vi "Convert SPI Data to Numbers.vi"(0 "Data In":bool[](array[boolean])) -> (1 "IBP Data":T1, 2 "ECG Data":T2)   [LabVIEW 2016]
uses:
  ECG Data.ctl
  IBP Data.ctl
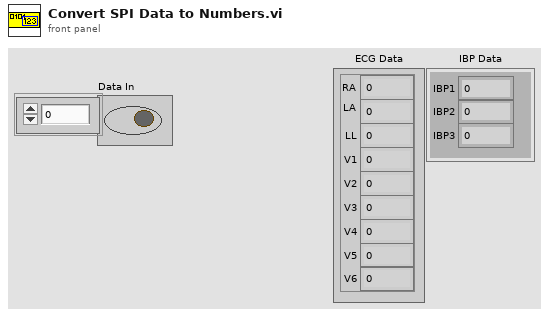
[diagram p1: front panel]
types:
  T1 = typedef "IBP Data.ctl" = cluster{"IBP1":fxp<+/-,16,16>, "IBP2":fxp<+/-,16,16>, "IBP3":fxp<+/-,16,16>}
  T2 = typedef "ECG Data.ctl" = cluster{"RA":fxp<+/-,16,16>, "LA":fxp<+/-,16,16>, "LL":fxp<+/-,16,16>, "V1":fxp<+/-,16,16>, "V2":fxp<+/-,16,16>, "V3":fxp<+/-,16,16>, "V4":fxp<+/-,16,16>, "V5":fxp<+/-,16,16>, "V6":fxp<+/-,16,16>}
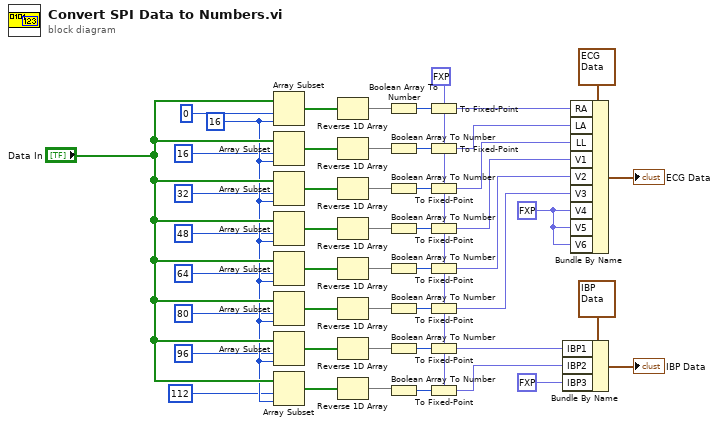
[diagram p0: block diagram]
diagram:
  w9 = fxp<+/-,16,16> 0.0 ("V4")
  w3 = fxp<+/-,16,16> 0.0 ("fixed-point type")
  w24 = 16 ("length")
  n1 = Array Subset(array="Data In", index=0, length=w24) -> (w34:bool[])
  n2 = Array Subset(array="Data In", index=16, length=w24) -> (w35:bool[])
  n3 = Array Subset(array="Data In", index=32, length=w24) -> (w36:bool[])
  n4 = Array Subset(array="Data In", index=48, length=w24) -> (w37:bool[])
  n5 = Array Subset(array="Data In", index=64, length=w24) -> (w38:bool[])
  n6 = Array Subset(array="Data In", index=80, length=w24) -> (w39:bool[])
  n7 = Array Subset(array="Data In", index=96, length=w24) -> (w40:bool[])
  n8 = Array Subset(array="Data In", index=112, length=w24) -> (w41:bool[])
  n9 = Reverse 1D Array(array=w34) -> (reversed array=w26:bool[])
  n10 = Reverse 1D Array(array=w35) -> (reversed array=w33:bool[])
  n11 = Reverse 1D Array(array=w36) -> (reversed array=w27:bool[])
  n12 = Reverse 1D Array(array=w37) -> (reversed array=w32:bool[])
  n13 = Reverse 1D Array(array=w38) -> (reversed array=w28:bool[])
  n14 = Reverse 1D Array(array=w39) -> (reversed array=w31:bool[])
  n15 = Reverse 1D Array(array=w40) -> (reversed array=w29:bool[])
  n16 = Reverse 1D Array(array=w41) -> (reversed array=w30:bool[])
  n17 = Boolean Array To Number(Boolean array=w26) -> (number=w43:i16)
  n18 = Boolean Array To Number(Boolean array=w33) -> (number=w44:i16)
  n19 = Boolean Array To Number(Boolean array=w27) -> (number=w45:i16)
  n20 = Boolean Array To Number(Boolean array=w32) -> (number=w46:i16)
  n21 = Boolean Array To Number(Boolean array=w28) -> (number=w47:i16)
  n22 = Boolean Array To Number(Boolean array=w31) -> (number=w48:i16)
  n23 = Boolean Array To Number(Boolean array=w29) -> (number=w7:i16)
  n24 = Boolean Array To Number(Boolean array=w30) -> (number=w6:i16)
  n25 = To Fixed-Point(fixed-point type=w3, number=w43) -> (fixed-point=w15:fxp<+/-,16,16>)
  n26 = To Fixed-Point(fixed-point type=w3, number=w44) -> (fixed-point=w14:fxp<+/-,16,16>)
  n27 = To Fixed-Point(fixed-point type=w3, number=w45) -> (fixed-point=w13:fxp<+/-,16,16>)
  n28 = To Fixed-Point(fixed-point type=w3, number=w46) -> (fixed-point=w12:fxp<+/-,16,16>)
  n29 = To Fixed-Point(fixed-point type=w3, number=w47) -> (fixed-point=w11:fxp<+/-,16,16>)
  n30 = To Fixed-Point(fixed-point type=w3, number=w48) -> (fixed-point=w10:fxp<+/-,16,16>)
  n31 = To Fixed-Point(fixed-point type=w3, number=w7) -> (fixed-point=w5:fxp<+/-,16,16>)
  n32 = To Fixed-Point(fixed-point type=w3, number=w6) -> (fixed-point=w4:fxp<+/-,16,16>)
  n33 = Bundle By Name(cluster=T1 {"IBP1"=0.0, "IBP2"=0.0, "IBP3"=0.0} ("IBP Data"), "IBP1"=w5, "IBP2"=w4, "IBP3"=fxp<+/-,16,16> 0.0) -> (→"IBP Data":T1)
  n34 = Bundle By Name(cluster=T2 {"RA"=0.0, "LA"=0.0, "LL"=0.0, "V1"=0.0, "V2"=0.0, "V3"=0.0, "V4"=0.0, "V5"=0.0, "V6"=0.0} ("ECG"), "RA"=w15, "LA"=w14, "LL"=w13, "V1"=w12, "V2"=w11, "V3"=w10, "V4"=w9, "V5"=w9, "V6"=w9) -> (→"ECG Data":T2)
